vi "EthernetTest.vi"() -> ()   [LabVIEW 2017]
panel:
  in  "write buffer 2":string
  in  "write buffer":string
  out "read buffer":string
  in  "VISA resource name":refnum<visa-resource-name>
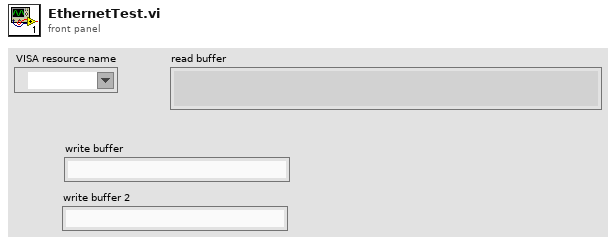
[diagram p1: front panel]
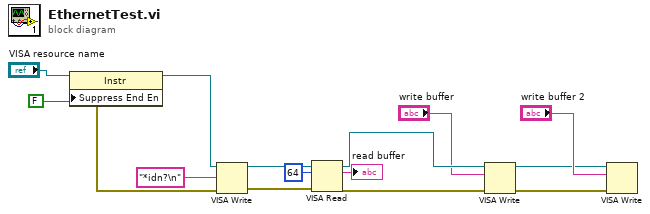
[diagram p0: block diagram]
diagram:
  n1 = property class="Instr"(reference="VISA resource name", "Suppress End En"=FALSE ("Message Based Settings:Send End Enable")) -> (reference out=w10:refnum<visa-resource-name>, error out=w9:errorcluster)  [unwired: 1 in]
  n2 = VISA Write(VISA resource name=w10, write buffer="*idn?\n", error in (no error)=w9) -> (VISA resource name out=w15:refnum<visa-resource-name>, error out=w14:errorcluster)  [unwired: 1 out]
  n3 = VISA Read(VISA resource name=w15, byte count=u32 64, error in (no error)=w14) -> (VISA resource name out=w6:refnum<visa-resource-name>, read buffer=→"read buffer":string, error out=w4:errorcluster)  [unwired: 1 out]
  n4 = VISA Write(VISA resource name=w6, write buffer="write buffer", error in (no error)=w4) -> (VISA resource name out=w2:refnum<visa-resource-name>, error out=w1:errorcluster)  [unwired: 1 out]
  n5 = VISA Write(VISA resource name=w2, write buffer="write buffer 2", error in (no error)=w1) -> ()  [unwired: 3 out]
